vi "DSF.Engine.Execution.Transfer.RT FIFO.Write.vi"(8 "error in (no error)":errorcluster, 9 "timeout in ms (0)":i32, 10 "Transfer":refnum<class "DSF.Engine.Execution.Transfer.lvclass">, 11 "Transfer FIFO in":T1) -> (0 "error out":errorcluster, 1 "timed out?":bool, 3 "Transfer FIFO out":T1)   [LabVIEW 2016, in "DSF.Engine.lvlib" / "DSF.Engine.Execution.Transfer.lvclass"]
uses:
  DSF.Engine.Execution.Transfer.lvclass
  DSF.Engine.Execution.Transfer.RT FIFO Ref.ctl
  DSF.Engine.Execution.Transfer.RT FIFO Data.ctl
  DSF.Engine.Execution.Transfer.lvclass/DSF.Engine.Execution.Transfer.ctl
  Submodules/Memory/Source/Classes/Pointer/Memory.Pointer.lvclass/Memory.Pointer.ctl
  Submodules/Memory/Source/Classes/Pointer/Memory.Pointer.Object To Block Descriptor.vi
  DSF.Engine.Execution.Transfer.Get Buffer.vi
  DSF.Engine.Execution.Transfer.Get ID.vi
  Submodules/Memory/Source/Classes/Pointer/Memory.Pointer.Get Address.vi
  Submodules/Memory/Source/Classes/Pointer/Memory.Pointer.Get Size.vi
  Buffer/DSF.Engine.Memory.Buffer.lvclass
  C:/Git/SourceTree/DSF/Source/Submodules/Memory/Source/Classes/Pointer/Memory.Pointer.lvclass
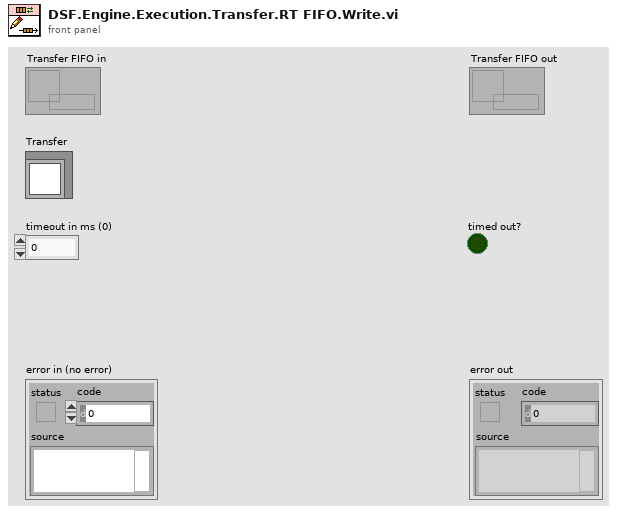
[diagram p1: front panel]
types:
  T1 = typedef "DSF.Engine.lvlib/DSF.Engine.Execution.Transfer.lvclass/DSF.Engine.Execution.Transfer.RT FIFO Ref.ctl" = refnum<k33>
  T2 = typedef "DSF.Engine.lvlib/DSF.Engine.Execution.Transfer.lvclass/DSF.Engine.Execution.Transfer.RT FIFO Data.ctl" = cluster{"ID":i32, "Buffer Descriptor":cluster{"address":u64, "size":u64}}
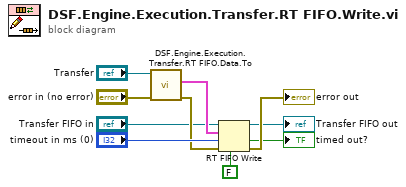
[diagram p0: block diagram]
diagram:
  n1 = call "DSF.Engine.Execution.Transfer.RT FIFO.Data.To.vi"("error in (no error)"="error in (no error)", "Transfer in"="Transfer") -> ("error out"=w6:errorcluster, "Transfer Data"=w5:T2)  [unwired: 7 in, 1 out]
  n2 = RT FIFO Write(0:"Transfer FIFO in", 1:w5, 2:"timeout in ms (0)", 3:w6, 5:FALSE ("overwrite on timeout (T)")) -> (8:→"Transfer FIFO out":T1, 10:→"timed out?":bool, 11:→"error out":errorcluster)  [unwired: 1 out]
